vi "UHR-Fleezers Control (host) - 12.2.vi"() -> ()   [LabVIEW 2012] (continued)
      event "Green FB Setpoint (mV)", "Green FB Gains", "Green FB On/Off", "Current When FB OFF (%)", "Green int current ON count adj": Value Change {
        n2009 = event-data() -> ()  [unwired: 7 out]
        n2010 = local read "Green FB Setpoint (mV)"() -> (w3377:dbl)
        n2011 = Multiply(x=w3377, y=3.2767) -> (x*y=w3376:dbl)
        n2012 = local read "Current When FB OFF (%)"() -> (w3380:dbl)
        n2013 = Multiply(x=w3380, y=655.35) -> (x*y=w3381:dbl)
        n2014 = To Unsigned Word Integer(number=w3381) -> (unsigned 16bit integer=w3379:u16)
        n2015 = local read "Green int current ON count adj"() -> (w3383:u32)
        n2016 = local read "Green Laser ON/Interlacing"() -> (w3374:bool)
        n2017 = local read "Laser interlacing mode"() -> (w3373:enum32{"Laser ON", "Laser OFF", "Interlace"})
        n2018 = local read "Green FB Gains"() -> (w3370:T9)
        n2019 = local read "Green FB On/Off"() -> (w3384:bool)
        n2020 = Equal?(x=w3373, y=enum32{"Laser ON", "Laser OFF", "Interlace"}."Interlace") -> (x = y?=w3371:bool)
        n2021 = Unbundle By Name(w3370) -> ("proportional gain (Kc)"=w3369:i16, "integral gain (Kc*Ts/Ti)"=w3368:i16, "derivative gain (Kc*Td/Ts)"=w3367:i16)
        n2022 = Compound Arithmetic op=AND(w3371, w3384, w3374) -> (w3375:bool)
        n2023 = xnode "Read/Write Control"("FPGA VI Reference In"=w3387, "error in"=w3386, "Green FB Setpoint"=w3376, "Green FB On/Off"=w3375, "Current Out"=w3379, "Green int current ON count adj"=w3383, "P3"=w3369, "I3"=w3368, "D3"=w3367) -> ("error out"=w3385:errorcluster)  [unwired: 1 out]
      }
      event "Red FB Setpoint (mV)", "Red FB Gains", "Red FB On/Off", "Current When RI FB OFF (%)", "Red int current ON count adj": Value Change {
        n2024 = event-data() -> ()  [unwired: 7 out]
        n2025 = local read "Red FB Setpoint (mV)"() -> (w3399:dbl)
        n2026 = Multiply(x=w3399, y=3.2767) -> (x*y=w3398:dbl)
        n2027 = local read "Current When RI FB OFF (%)"() -> (w3388:dbl)
        n2028 = Multiply(x=w3388, y=655.35) -> (x*y=w3402:dbl)
        n2029 = To Unsigned Word Integer(number=w3402) -> (unsigned 16bit integer=w3401:u16)
        n2030 = local read "Red int current ON count adj"() -> (w3404:u32)
        n2031 = local read "Red Laser ON/Interlacing"() -> (w3396:bool)
        n2032 = local read "Laser interlacing mode"() -> (w3395:enum32{"Laser ON", "Laser OFF", "Interlace"})
        n2033 = local read "Red FB Gains"() -> (w3392:T9)
        n2034 = local read "Red FB On/Off"() -> (w3405:bool)
        n2035 = Equal?(x=w3395, y=enum32{"Laser ON", "Laser OFF", "Interlace"}."Interlace") -> (x = y?=w3393:bool)
        n2036 = Unbundle By Name(w3392) -> ("proportional gain (Kc)"=w3391:i16, "integral gain (Kc*Ts/Ti)"=w3390:i16, "derivative gain (Kc*Td/Ts)"=w3389:i16)
        n2037 = Compound Arithmetic op=AND(w3393, w3405, w3396) -> (w3397:bool)
        n2038 = xnode "Read/Write Control"("FPGA VI Reference In"=w3408, "error in"=w3407, "Red FB Setpoint"=w3398, "Red FB On/Off"=w3397, "RI Current Out"=w3401, "Red int current ON count adj"=w3404, "P4"=w3391, "I4"=w3390, "D4"=w3389) -> ("error out"=w3406:errorcluster)  [unwired: 1 out]
      }
      event "Laser interlacing mode", "Green Laser ON/Interlacing", "Red Laser ON/Interlacing": Value Change {
        n2039 = event-data() -> ()  [unwired: 7 out]
        n2040 = local write "Green Laser ON/OFF"("Green Laser ON/Interlacing") -> ()
        n2041 = local write "Red Laser ON/OFF"("Red Laser ON/Interlacing") -> ()
        n2042 = case shown="True" "Green Laser ON/Interlacing" {
          tunnel: "Laser interlacing mode" -> [_ w3432]
          tunnel: [enum32{"Laser ON", "Laser OFF", "Interlace"}."Laser OFF" ("Green laser mode") w3432] -> w3415
          tunnel: [FALSE w3428] -> w3414
          frame False {
          }
          frame True {
            n2043 = local read "Green FB On/Off"() -> (w3429:bool)
            n2044 = Equal?(x=w3432, y=enum32{"Laser ON", "Laser OFF", "Interlace"}."Interlace") -> (x = y?=w3430:bool)
            n2045 = And(x=w3430, y=w3429) -> (x .and. y?=w3428:bool)
          }
        }
        n2046 = case shown="True" "Red Laser ON/Interlacing" {
          tunnel: "Laser interlacing mode" -> [_ w3425]
          tunnel: [enum32{"Laser ON", "Laser OFF", "Interlace"}."Laser OFF" ("Green laser mode") w3425] -> w3410
          tunnel: [FALSE w3421] -> w3409
          frame False {
          }
          frame True {
            n2047 = local read "Red FB On/Off"() -> (w3422:bool)
            n2048 = Equal?(x=w3425, y=enum32{"Laser ON", "Laser OFF", "Interlace"}."Interlace") -> (x = y?=w3423:bool)
            n2049 = And(x=w3423, y=w3422) -> (x .and. y?=w3421:bool)
          }
        }
        n2050 = xnode "Read/Write Control"("FPGA VI Reference In"=w3418, "error in"=w3416, "Operating Mode"=w3415, "Operating Mode 2"=w3415, "Green FB On/Off"=w3414, "Red Laser Operating Mode"=w3410, "RI Operating Mode 2"=w3410, "Red FB On/Off"=w3409) -> ("error out"=w3417:errorcluster)  [unwired: 1 out]
      }
      event "Green Laser ON/OFF": Value Change {
        n2051 = event-data() -> ()  [unwired: 7 out]
        n2052 = property on="Green Laser ON/Interlacing" class="Bool (strict)"("Val(Sgnl)"="Green Laser ON/OFF") -> ()  [unwired: 2 in, 2 out]
      }
      event "Red Laser ON/OFF": Value Change {
        n2053 = event-data() -> ()  [unwired: 7 out]
        n2054 = property on="Red Laser ON/Interlacing" class="Bool (strict)"("Val(Sgnl)"="Red Laser ON/OFF") -> ()  [unwired: 2 in, 2 out]
      }
      event "Test ttrig": Value Change {
        n2055 = event-data() -> ()  [unwired: 7 out]
        n2056 = xnode "Read/Write Control"("FPGA VI Reference In"=w3438, "error in"=w3437, "TTrig?"=TRUE) -> ("error out"=w3436:errorcluster)  [unwired: 1 out]
      }
      event "Neg. TTrig FPGA": Value Change {
        n2057 = event-data() -> ()  [unwired: 7 out]
        n2058 = xnode "Read/Write Control"("FPGA VI Reference In"=w3442, "error in"=w3441, "TTrig Negate Pos"="Neg. TTrig FPGA") -> ()  [unwired: 2 out]
      }
      event "- phase (APD 1 Gate)", "+ phase (APD 1 Gate)": Value Change {
        n2059 = event-data() -> ()  [unwired: 7 out]
        n2060 = local read "Phase Adj. (APD 1 Gate)"() -> (w3443:i16)
        n2061 = Negate(x=w3443) -> (-x=w3451:i16)
        n2062 = Select(t=w3451, s="- phase (APD 1 Gate)", f=w3443) -> (s? t:f=w3450:i16)
        n2063 = Or(x="- phase (APD 1 Gate)", y="+ phase (APD 1 Gate)") -> (x .or. y?=w3446:bool)
        n2064 = xnode "Read/Write Control"("FPGA VI Reference In"=w3453, "error in"=w3452, "Phase count adjustment (APD 1 Gate)"=w3450) -> ("FPGA VI Reference Out"=w3448:T19, "error out"=w3449:errorcluster)
        n2065 = xnode "Read/Write Control"("FPGA VI Reference In"=w3448, "error in"=w3449, "+ phase (APD 1 Gate)"=w3446) -> ("error out"=w3447:errorcluster)  [unwired: 1 out]
      }
      event "+ phase (APD 2 Gate)", "- phase (APD 2 Gate)": Value Change {
        n2066 = event-data() -> ()  [unwired: 7 out]
        n2067 = local read "Phase Adj. (APD 2 Gate)"() -> (w3454:i16)
        n2068 = Negate(x=w3454) -> (-x=w3462:i16)
        n2069 = Select(t=w3462, s="- phase (APD 2 Gate)", f=w3454) -> (s? t:f=w3461:i16)
        n2070 = Or(x="- phase (APD 2 Gate)", y="+ phase (APD 2 Gate)") -> (x .or. y?=w3457:bool)
        n2071 = xnode "Read/Write Control"("FPGA VI Reference In"=w3464, "error in"=w3463, "Phase count adjustment (APD 2 Gate)"=w3461) -> ("FPGA VI Reference Out"=w3459:T19, "error out"=w3460:errorcluster)
        n2072 = xnode "Read/Write Control"("FPGA VI Reference In"=w3459, "error in"=w3460, "+ phase (APD 2 Gate)"=w3457) -> ("error out"=w3458:errorcluster)  [unwired: 1 out]
      }
      event "Phase Adj. (APD Acq)", "+ phase (APD Acq)", "- phase (APD Acq)": Value Change {
        n2073 = event-data() -> ()  [unwired: 7 out]
        n2074 = local read "Phase Adj. (APD Acq)"() -> (w3467:i16)
        n2075 = Negate(x=w3467) -> (-x=w3473:i16)
        n2076 = Select(t=w3473, s="+ phase (APD Acq)", f=w3467) -> (s? t:f=w3472:i16)
        n2077 = Or(x="+ phase (APD Acq)", y="- phase (APD Acq)") -> (x .or. y?=w3468:bool)
        n2078 = xnode "Read/Write Control"("FPGA VI Reference In"=w3475, "error in"=w3474, "Phase Count Adjustment (APD Acq)"=w3472) -> ("FPGA VI Reference Out"=w3470:T19, "error out"=w3471:errorcluster)
        n2079 = xnode "Read/Write Control"("FPGA VI Reference In"=w3470, "error in"=w3471, "+ phase (APD Acq)"=w3468) -> ("error out"=w3469:errorcluster)  [unwired: 1 out]
      }
      event "Phase adj. (GI)", "+ phase (GI)", "- phase (GI)", "Phase adj. (GI) 2", "+ phase (GI) 2", "- phase (GI) 2", "Phase adj. (RI)", "+ phase (RI)", "- phase (RI)", "Phase adj. (RI) 2", "+ phase (RI) 2", "- phase (RI) 2", "Phase adj. (Green FB)", "+ phase (Green FB)", "- phase (Green FB)", "Phase adj. (RI FB)", "+ phase (RI FB)", "- phase (RI FB)": Value Change {
        n2080 = event-data() -> ()  [unwired: 7 out]
        n2081 = Or(x="+ phase (GI)", y="- phase (GI)") -> (x .or. y?=w3509:bool)
        n2082 = Negate(x="Phase adj. (GI)") -> (-x=w3514:i16)
        n2083 = Select(t=w3514, s="+ phase (GI)", f="Phase adj. (GI)") -> (s? t:f=w3513:i16)
        n2084 = Or(x="+ phase (GI) 2", y="- phase (GI) 2") -> (x .or. y?=w3500:bool)
        n2085 = Negate(x="Phase adj. (GI) 2") -> (-x=w3505:i16)
        n2086 = Select(t=w3505, s="+ phase (GI) 2", f="Phase adj. (GI) 2") -> (s? t:f=w3501:i16)
        n2087 = Negate(x="Phase adj. (RI)") -> (-x=w3499:i16)
        n2088 = Or(x="+ phase (RI)", y="- phase (RI)") -> (x .or. y?=w3495:bool)
        n2089 = Select(t=w3499, s="+ phase (RI)", f="Phase adj. (RI)") -> (s? t:f=w3494:i16)
        n2090 = Negate(x="Phase adj. (RI) 2") -> (-x=w3493:i16)
        n2091 = Or(x="+ phase (RI) 2", y="- phase (RI) 2") -> (x .or. y?=w3482:bool)
        n2092 = Select(t=w3493, s="+ phase (RI) 2", f="Phase adj. (RI) 2") -> (s? t:f=w3489:i16)
        n2093 = Or(x="+ phase (Green FB)", y="- phase (Green FB)") -> (x .or. y?=w3483:bool)
        n2094 = Negate(x="Phase adj. (Green FB)") -> (-x=w3488:i16)
        n2095 = Select(t=w3488, s="+ phase (Green FB)", f="Phase adj. (Green FB)") -> (s? t:f=w3484:i16)
        n2096 = Or(x="+ phase (RI FB)", y="- phase (RI FB)") -> (x .or. y?=w3476:bool)
        n2097 = Negate(x="Phase adj. (RI FB)") -> (-x=w3481:i16)
        n2098 = Select(t=w3481, s="+ phase (RI FB)", f="Phase adj. (RI FB)") -> (s? t:f=w3477:i16)
        n2099 = xnode "Read/Write Control"("FPGA VI Reference In"=w3516, "error in"=w3515, "Phase count adjustment (GI)"=w3513, "Phase count adjustment (GI) 2"=w3501, "Phase count adjustment (RI)"=w3494, "Phase count adjustment (RI) 2"=w3489, "Phase count adjustment (Green FB)"=w3484, "Phase count adjustment (Red FB)"=w3477) -> ("FPGA VI Reference Out"=w3511:T19, "error out"=w3512:errorcluster)
        n2100 = xnode "Read/Write Control"("FPGA VI Reference In"=w3511, "error in"=w3512, "+ phase (GI)"=w3509, "+ phase (GI) 2"=w3500, "+ phase (RI)"=w3495, "+ phase (RI) 2"=w3482, "+ phase (Green FB)"=w3483, "+ phase (Red FB)"=w3476) -> ("error out"=w3510:errorcluster)  [unwired: 1 out]
      }
      event "Invert APD Gate", "APD Gate ON Count", "APD Gate OFF Count", "APD Gate", "APD Integration Time (s)", "APD 1 AO Mult.", "APD 2 AO Mult.", "Duty Cycles (ON one out of N cycles)": Value Change {
        n2101 = event-data() -> ()  [unwired: 7 out]
        n2102 = Add(x="Interlace Frequency, ON count", y="Interlace Frequency, OFF count") -> (x+y=w3521:u32)
        n2103 = Add(x="APD Gate ON Count", y="APD Gate OFF Count") -> (x+y=w3533:u32)
        n2104 = Multiply(x="Duty Cycles (ON one out of N cycles)", y=w3521) -> (x*y=w3517:u32)
        "Green FB Count" <- w3517
        "Red FB Count" <- w3517
        n2105 = Subtract(x=w3517, y="Interlace Frequency, ON count") -> (x-y=w3520:u32)
        n2106 = Multiply(x=w3533, y="Duty Cycles (ON one out of N cycles)") -> (x*y=w3532:u32)
        n2107 = Subtract(x=w3532, y="APD Gate ON Count") -> (x-y=w3531:u32)
        n2108 = local read "DMA Update Period (s)"() -> (w3534:dbl)
        n2109 = Multiply(x="APD Integration Time (s)", y=40000000.0) -> (x*y=w3539:dbl)
        n2110 = Reciprocal(x="APD Integration Time (s)") -> (1/x=→"APD Acq Rate (Hz)":dbl)
        n2111 = To Unsigned Long Integer(number=w3539) -> (unsigned 32bit integer=w3523:u32)
        "APD Int. Count" <- w3523
        n2112 = Divide(x=w3534, y="APD Integration Time (s)") -> (x/y=w3537:dbl)
        n2113 = Multiply(x=2.0, y=w3537) -> (x*y=w3536:dbl)
        n2114 = local write "APD Samples/FIFO Acq."(w3537) -> ()
        n2115 = xnode "Read/Write Control"("FPGA VI Reference In"=w3543, "error in"=w3542, "Invert APD Gate"="Invert APD Gate", "APD Gate ON Count"="APD Gate ON Count", "APD Gate OFF Count"=w3531, "APD Acq Rate Count"=w3523, "APD Gate Operating Mode"="APD Gate", "APD 1 AO scale factor"="APD 1 AO Mult.", "APD 2 AO scale factor"="APD 2 AO Mult.", "Green interlace ON count"="Interlace Frequency, ON count", "Green interlace OFF count"=w3520, "Green interlace ON count 2"="Interlace Frequency, ON count", "Green interlace OFF count 2"=w3520, "Green FB Count"=w3517, "Red interlace ON count"="Interlace Frequency, ON count", "Red interlace OFF count"="Interlace Frequency, OFF count", "Red FB Count"=w3517, "Red interlace ON count 2"="Interlace Frequency, ON count", "Red interlace OFF count 2"="Interlace Frequency, OFF count") -> ("error out"=w3541:errorcluster)  [unwired: 1 out]
        n2116 = local write "APD Elements/DMA read"(w3536) -> ()
      }
      event "Number of F/B Scans (AOD)", "Scan Speed (nm/s)", "Scan BD", "Initial delta (MHz)", "Step Size (nm)", "Scan Range (nm)": Value Change {
        w3605 = 123.0  # AOM cal (nm/MHz)
        n2117 = event-data() -> ()  [unwired: 7 out]
        n2118 = local read "BD 1 Frequency 1 (MHz)"() -> (w3588:dbl)
        n2119 = local read "AOM X Cal (nm/MHz)"() -> (w3580:dbl)
        n2120 = local read "X RF Frequency Limits (MHz)"() -> (w3592:T16)
        n2121 = local read "Y RF Frequency Limits (MHz)"() -> (w3589:T16)
        n2122 = local read "BD 2 Frequency 1 (MHz)"() -> (w3594:dbl)
        n2123 = Negate(x="Scan Range (nm)") -> (-x=w3558:dbl)
        n2124 = Divide(x=w3558, y=w3580) -> (x/y=w3562:dbl)
        n2125 = Select(t=w3592, s="Scan BD", f=w3589) -> (s? t:f=w3591:T16)
        n2126 = Select(t=w3588, s="Scan BD", f=w3594) -> (s? t:f=w3593:dbl)
        n2127 = Unbundle By Name(w3591) -> ("Maximum"=w3600:dbl, "Minimum"=w3599:dbl)
        n2128 = Add(x=w3562, y=w3593) -> (x+y=w3597:dbl)
        n2129 = Divide(x=w3558, y="Step Size (nm)") -> (x/y=w3577:dbl)
        n2130 = Divide(x="Step Size (nm)", y=w3580) -> (x/y=w3586:dbl)
        n2131 = Absolute Value(x=w3577) -> (abs(x)=w3561:dbl)
        n2132 = Sign(1:w3558) -> (0:w3559:dbl)
        n2133 = In Range and Coerce(upper limit=w3600, x=w3597, lower limit=w3599) -> (coerced(x)=w3596:dbl, In Range?=w3598:bool)
        n2134 = To Unsigned Quad Integer(1:w3561) -> (0:w3576:u64)
        "Scan steps (AOD)" <- w3576
        n2135 = call "IR AOM freq to word.vi"("Frequency In (MHz)"=w3586) -> ("Frequency Word Out (double)"=w3583:dbl)
        n2136 = Multiply(x=w3559, y=w3583) -> (x*y=w3560:dbl)
        n2137 = Subtract(x=w3597, y=w3596) -> (x-y=w3595:dbl)
        n2138 = To Quad Integer(1:w3560) -> (0:w3582:i64)
        "Incr. int (AOD)" <- w3582
        n2139 = Subtract(x=w3562, y=w3595) -> (x-y=w3581:dbl)
        "Scan Range (MHz)" <- w3581
        n2140 = Select(t=w3562, s=w3598, f=w3581) -> (s? t:f=w3601:dbl)
        n2141 = Multiply(x=w3581, y=w3580) -> (x*y=w3579:dbl)
        n2142 = Decrement(x=w3576) -> (x-1=w3629:u64)
        n2143 = Negate(x=w3579) -> (-x=w3575:dbl)
        n2144 = local write "Scan Range (nm)"(w3575) -> ()
        n2145 = Divide(x=w3601, y=w3629) -> (x/y=w3585:dbl)
        "Scan Increment (MHz)" <- w3585
        n2146 = call "IR AOM freq to word.vi"("Frequency In (MHz)"=w3585) -> ("Frequency Word Out (double)"=w3584:dbl)
        n2147 = Divide(x="Step Size (nm)", y="Scan Speed (nm/s)") -> (x/y=w3572:dbl)
        n2148 = To Quad Integer(1:w3584) -> ()  [unwired: 1 out]
        n2149 = local read "Number Interlace Sets"() -> (w3556:u8)
        n2150 = local read "AI Count (ticks)"() -> (w3557:u32)
        n2151 = local read "Total Counts (ticks)"() -> (w3555:u32)
        n2152 = local read "# Samples/trap"() -> (w3587:u32)
        n2153 = Multiply(x=w3557, y=w3556) -> (x*y=w3554:u32)
        n2154 = Divide(x=w3555, y=w3554) -> (x/y=w3553:dbl)
        n2155 = Select(t=w3588, s="Scan BD", f=w3594) -> (s? t:f=w3626:dbl)
        "Initial freq. (MHz)" <- w3626
        n2156 = Add(x=w3601, y=w3626) -> (x+y=→"Final freq. (MHz)":dbl)
        n2157 = Divide(x=w3555, y=40000000.0) -> (x/y=w3571:dbl)
        n2158 = Divide(x=w3572, y=w3571) -> (x/y=w3570:dbl)
        n2159 = To Unsigned Quad Integer(1:w3570) -> (0:w3545:u64)
        n2160 = Quotient & Remainder(x=w3545, y=u64 2) -> (x-y*floor(x/y)=w3549:u64)  [unwired: 1 out]
        n2161 = Equal?(x=w3549, y=u64 0) -> (x = y?=w3547:bool)
        n2162 = Decrement(x=w3545) -> (x-1=w3546:u64)
        n2163 = Select(t=w3545, s=w3547, f=w3546) -> (s? t:f=w3544:u64)
        "Cycles/step (AOD)" <- w3544
        n2164 = xnode "Read/Write Control"("FPGA VI Reference In"=w3637, "error in"=w3636, "Scan steps"=w3576, "Number of scans"="Number of F/B Scans (AOD)", "Cycles per step"=w3544, "Scan freq.  increment"=w3582, "Scan BD"="Scan BD") -> ("error out"=w3635:errorcluster)  [unwired: 1 out]
        n2165 = Multiply(x=w3576, y=w3544) -> (x*y=w3630:u64)
        n2166 = Multiply(x=w3630, y=u64 2) -> (x*y=w3552:u64)
        n2167 = Multiply(x=w3553, y=w3552) -> (x*y=w3551:dbl)
        "Data points/scan (f/b)" <- w3551
        n2168 = Multiply(x=w3551, y="Number of F/B Scans (AOD)") -> (x*y=w3633:dbl)
        "Data points/scans" <- w3633
        n2169 = Divide(x=w3633, y=w3587) -> (x/y=→"N sets should be saved":dbl)
        n2170 = Multiply(x=w3630, y=w3571) -> (x*y=w3569:dbl)
        "Time/Scan (s) (AOD)" <- w3569
        n2171 = Select(t=w3601, s="Scan BD", f=0.0) -> (s? t:f=w3627:dbl)
        n2172 = Select(t=0.0, s="Scan BD", f=w3601) -> (s? t:f=w3623:dbl)
        n2173 = local read "BD 2 Frequency 2 (MHz)"() -> (w3619:dbl)
        n2174 = local read "BD 1 Frequency 2 (MHz)"() -> (w3622:dbl)
        n2175 = Add(x=w3623, y=w3594) -> (x+y=w3620:dbl)
        n2176 = Add(x=w3588, y=w3627) -> (x+y=w3621:dbl)
        n2177 = Multiply(x=w3569, y=2.0) -> (x*y=w3568:dbl)
        n2178 = Multiply(x=w3568, y="Number of F/B Scans (AOD)") -> (x*y=w3565:dbl)
        n2179 = Divide(x=w3565, y=60.0) -> (x/y=→"Time to Finish All (min)":dbl)
        n2180 = Add(x="Trap 2 Bead Size (nm)", y="Trap 1 Bead Size (nm)") -> (x+y=w3609:dbl)
        n2181 = Divide(x=w3609, y=2.0) -> (x/y=w3603:dbl)
        n2182 = local read "Initial delta (MHz)"() -> (w3606:dbl)
        n2183 = Subtract(x=w3620, y=w3619) -> (x-y=w3617:dbl)
        n2184 = Subtract(x=w3621, y=w3622) -> (x-y=w3618:dbl)
        n2185 = Square(x=w3617) -> (x^2=w3616:dbl)
        n2186 = Square(x=w3618) -> (x^2=w3615:dbl)
        n2187 = Add(x=w3615, y=w3616) -> (x+y=w3614:dbl)
        n2188 = Square Root(x=w3614) -> (sqrt(x)=w3613:dbl)
        "Final delta (MHz)" <- w3613
        n2189 = Multiply(x=w3605, y=w3613) -> (x*y=w3612:dbl)
        n2190 = Multiply(x=w3606, y=w3605) -> (x*y=w3604:dbl)
        n2191 = Subtract(x=w3604, y=w3603) -> (x-y=→"Initial sep (nm)":dbl)
        n2192 = Subtract(x=w3612, y=w3603) -> (x-y=→"Final sep (nm)":dbl)
      }
      event "Freq or Amp switch first", "Swap F1 and F2", "Freq switch delay", "Amp switch delay": Value Change {
        n2193 = event-data() -> ()  [unwired: 7 out]
        n2194 = local read "Amp switch delay"() -> (w3638:u16)
        n2195 = local read "Swap F1 and F2"() -> (w3639:bool)
        n2196 = xnode "Read/Write Control"("FPGA VI Reference In"=w3642, "error in"=w3641, "Swap F1 and F2"=w3639, "Amp switch delay"=w3638) -> ("error out"=w3640:errorcluster)  [unwired: 1 out]
      }
      event "Scan steps (MCL)", "Number of scans (MCL)", "Scan Range (V)\n(of steps)", "2D or 1D Scan", "N APD Samp/step", "Fast Scan Dir", "Continuous MCL Scanning", "Scan lines (y)": Value Change {
        w3644 = 32767.0 ("y")
        n2197 = event-data() -> ()  [unwired: 7 out]
        n2198 = Select(t="Scan lines (y)", s="2D or 1D Scan", f="Number of scans (MCL)") -> (s? t:f=w3649:u64)
        n2199 = Decrement(x="Scan steps (MCL)") -> (x-1=w3665:u64)
        n2200 = Divide(x="Scan Range (V)\n(of steps)", y=w3665) -> (x/y=w3664:dbl)
        "Desired Scan Incr (V)" <- w3664
        n2201 = local read "APD Integration Time (s)"() -> (w3657:dbl)
        n2202 = Multiply(x=w3664, y=w3644) -> (x*y=w3673:dbl)
        n2203 = Divide(x=w3673, y=10.0) -> (x/y=w3663:dbl)
        "Desired incr (int)" <- w3663
        n2204 = local read "Update Count (MCL)"() -> (w3669:u32)
        n2205 = Round Toward -Infinity(1:w3663) -> (0:w3672:dbl)
        n2206 = To Word Integer(number=w3672) -> (16bit integer=w3647:i16)
        "Actual Incr. int (MCL)" <- w3647
        n2207 = Multiply(x=w3657, y=40000000.0) -> (x*y=w3670:dbl)
        n2208 = Divide(x=w3670, y=w3669) -> (x/y=w3668:dbl)
        n2209 = Multiply(x=i16 10, y=w3647) -> (x*y=w3645:i16)
        n2210 = Multiply(x="N APD Samp/step", y=w3668) -> (x*y=w3667:dbl)
        "Cycles/step (MCL)" <- w3667
        n2211 = Divide(x=w3645, y=w3644) -> (x/y=→"Actual MCL Inc (V)":dbl)
        n2212 = Multiply(x="N APD Samp/step", y="Scan steps (MCL)") -> (x*y=w3659:dbl)
        n2213 = local read "APD Samples/FIFO Acq."() -> (w3656:dbl)
        n2214 = Multiply(x=w3659, y=u64 2) -> (x*y=w3658:dbl)
        "Data points/scan (f+b)" <- w3658
        n2215 = Multiply(x=w3658, y=w3649) -> (x*y=w3676:dbl)
        "Data points/scans (MCL)" <- w3676
        n2216 = Multiply(x=w3657, y=w3658) -> (x*y=w3650:dbl)
        "Time/f+b scan (s) (MCL)" <- w3650
        n2217 = Divide(x=w3676, y=w3656) -> (x/y=→"N sets should be saved (MCL)":dbl)
        n2218 = Multiply(x=w3650, y=w3649) -> (x*y=→"Total Time (s)":dbl)
        n2219 = Not(x="Fast Scan Dir") -> (.not. x?=w3654:bool)
        n2220 = xnode "Read/Write Control"("FPGA VI Reference In"=w3680, "error in"=w3679, "Scan steps (MCL)"="Scan steps (MCL)", "Number of scans (MCL)"=w3649, "Cycles per step (MCL)"=w3667, "Scan freq.  increment (MCL)"=w3647, "1D or 2D Scan?"="2D or 1D Scan", "MCL Scan Axis"=w3654, "Cont. Scan (MCL)"="Continuous MCL Scanning") -> ("error out"=w3678:errorcluster)  [unwired: 1 out]
      }
      event "Read Cal": Value Change {
        w3682 = 1000.0 ("y")
        n2221 = event-data() -> ()  [unwired: 7 out]
        n2222 = local read "Save file name"() -> (w3707:path)
        n2223 = local write "Read Cal"(FALSE ("Read Cal")) -> ()
        n2224 = Strip Path(path=w3707) -> (stripped path=w3706:path)  [unwired: 1 out]
        n2225 = Path To String(path=w3706) -> (string=w3705:string)
        n2226 = Concatenate Strings(w3705, "\\current.cal" ("string")) -> (w3703:string)
        n2227 = String To Path(string=w3703) -> (path=w3702:path)
        n2228 = Open/Create/Replace File(file path (use dialog)=w3702, operation (0:open)=T35."open", access (0:read/write)=enum16{"read/write", "read-only", "write-only"}."read-only") -> (refnum out=w3710:refnum<file>, error out=w3696:errorcluster)  [unwired: 1 in, 3 out]
        n2229 = Deny Access(4:w3696, 7:w3710) -> (0:w3695:errorcluster, 3:w3701:refnum<file>)  [unwired: 1 out]
        n2230 = Read from Binary File(5:0.0, 8:w3695, 9:T36."big-endian, network order" ("byte order (0:big-endian, network order)"), 10:-1 ("count (1)"), 11:w3701) -> (0:w3694:errorcluster, 2:w3692:dbl[], 3:w3697:refnum<file>)  [unwired: 2 out]
        n2231 = Array To Cluster(array=w3692) -> (cluster=w3691:T44)
        n2232 = Unbundle(w3691) -> ("[0]"=w3690:dbl, "[1]"=w3689:dbl, "[2]"=w3688:dbl, "[3]"=w3687:dbl, "[4]"=w3686:dbl, "[5]"=w3685:dbl)
        n2233 = Close File(refnum=w3697, error in=w3694) -> (error out=→"Read cal error":errorcluster)  [unwired: 1 out]
        n2234 = Multiply(x=w3685, y=w3682) -> (x*y=w3683:dbl)
        n2235 = local write "T2 kappa_x (pN/nm)"(w3687) -> ()
        n2236 = local write "T1 kappa_x (pN/nm)"(w3688) -> ()
        n2237 = local write "T1 alpha_x (nm/V)"(w3690) -> ()
        n2238 = local write "T2 alpha_x (nm/V)"(w3689) -> ()
        n2239 = Multiply(x=w3686, y=w3682) -> (x*y=w3684:dbl)
        n2240 = local write "T1 offset_x (mV)"(w3684) -> ()
        n2241 = local write "T2 offset_x (mV)"(w3683) -> ()
      }
      event "Abort MCL Scan": Value Change {
        n2242 = event-data() -> ()  [unwired: 7 out]
        n2243 = local write "MCL Scanning"(FALSE ("MCL Scanning")) -> ()
        n2244 = xnode "Read/Write Control"("FPGA VI Reference In"=w3715, "error in"=w3714, "Abort scan (MCL)"="Abort MCL Scan") -> ("error out"=w3713:errorcluster)  [unwired: 1 out]
      }
      event "Update Count (MCL)": Value Change {
        n2245 = event-data() -> ()  [unwired: 7 out]
        n2246 = xnode "Read/Write Control"("FPGA VI Reference In"=w3719, "error in"=w3718, "MCL count"="Update Count (MCL)") -> ("error out"=w3717:errorcluster)  [unwired: 1 out]
      }
      event "Phase adjust (MCL)", "+ phase (MCL)", "- phase (MCL)": Value Change {
        n2247 = event-data() -> ()  [unwired: 7 out]
        n2248 = Negate(x="Phase adjust (MCL)") -> (-x=w3728:i16)
        n2249 = Select(t=w3728, s="- phase (MCL)", f="Phase adjust (MCL)") -> (s? t:f=w3726:i16)
        n2250 = Or(x="- phase (MCL)", y="+ phase (MCL)") -> (x .or. y?=w3721:bool)
        n2251 = xnode "Read/Write Control"("FPGA VI Reference In"=w3730, "error in"=w3729, "Phase count adjustment (MCL)"=w3726) -> ("FPGA VI Reference Out"=w3722:T19, "error out"=w3723:errorcluster)
        n2252 = xnode "Read/Write Control"("FPGA VI Reference In"=w3722, "error in"=w3723, "+ phase (MCL)"=w3721) -> ("error out"=w3720:errorcluster)  [unwired: 1 out]
      }
      event "Abort AOD Scan": Value Change {
        n2253 = event-data() -> ()  [unwired: 7 out]
        n2254 = xnode "Read/Write Control"("FPGA VI Reference In"=w3734, "error in"=w3733, "Abort scan"="Abort AOD Scan") -> ("error out"=w3732:errorcluster)  [unwired: 1 out]
      }
      event "Continuous AOD Scanning": Value Change {
        n2255 = event-data() -> ()  [unwired: 7 out]
        n2256 = xnode "Read/Write Control"("FPGA VI Reference In"=w3738, "error in"=w3737, "Cont. Scan"="Continuous AOD Scanning") -> ("error out"=w3736:errorcluster)  [unwired: 1 out]
      }
      event "Index": Value Change {
        n2257 = event-data() -> ()  [unwired: 7 out]
        n2258 = call "Create new save file.vi"("Insert"="", "Ext"=".dat" ("string"), "Index In"="Index") -> ("Path Out"=→"Save file name":path, "Index Out"=w3739:dbl)
        "Save index" <- w3739
        n2259 = local write "Index"(w3739) -> ()
      }
      event "AO1", "AO2": Value Change {
        w3754 = 10.0 ("y")
        w3753 = 32767.0 ("y")
        n2260 = event-data() -> ()  [unwired: 7 out]
        n2261 = local read "AO2"() -> (w3752:dbl)
        n2262 = local read "AO1"() -> (w3749:dbl)
        n2263 = Multiply(x=w3749, y=w3753) -> (x*y=w3748:dbl)
        n2264 = Multiply(x=w3752, y=w3753) -> (x*y=w3751:dbl)
        n2265 = Divide(x=w3748, y=w3754) -> (x/y=w3747:dbl)
        n2266 = Divide(x=w3751, y=w3754) -> (x/y=w3750:dbl)
        n2267 = To Word Integer(number=w3747) -> (16bit integer=w3755:i16)
        n2268 = To Word Integer(number=w3750) -> (16bit integer=w3756:i16)
        n2269 = xnode "Read/Write Control"("FPGA VI Reference In"=w3746, "error in"=w3745, "AO1"=w3755, "AO2"=w3756) -> ("error out"=w3744:errorcluster)  [unwired: 1 out]
      }
      event "Inject Pump 1": Value Change {
        n2270 = event-data() -> ()  [unwired: 7 out]
        n2271 = local read "Use Harvard pumps\nfor beads (else Chemyx)"() -> (w3758:bool)
        n2272 = case shown="True" w3758 {
          tunnel: "Inject Pump 1" -> [w3762 w3800]
          tunnel: w3757 -> [_ w3801]
          frame False {
            n2273 = local read "Pump write delay (ms)"() -> (w3761:dbl)
            n2274 = local read "Chemyx Syringe Pump Serial Port"() -> (w3760:refnum<visa-resource-name>)
            n2275 = case shown="True" w3762 {
              tunnel: w3761 -> [w3768 w3782]
              tunnel: w3760 -> [w3765 w3781]
              frame False {
                n2276 = flat-sequence {
                  tunnel: w3765 -> [w3769]
                  tunnel: [w3769] -> w3766
                  tunnel: w3768 -> [_]
                  tunnel: [w3772] -> w3767
                  tunnel: w3766 -> [w3772]
                  tunnel: w3767 -> [w3773]
                  tunnel: [w3773] -> w3763
                  tunnel: [w3775] -> w3764
                  tunnel: w3763 -> [w3775]
                  tunnel: w3764 -> [w3777]
                  frame #0 {
                    n2277 = call "Write to pump.vi"("string"="enter pump1", "VISA resource name"=w3769) -> ()  [unwired: 1 out]
                  }
                  frame #1 {
                    n2278 = Wait (ms)(milliseconds to wait="Pump pause delay (ms)") -> ()  [unwired: 1 out]
                  }
                  frame #2 {
                    n2279 = call "Write to pump.vi"("string"="stop", "VISA resource name"=w3773) -> ()  [unwired: 1 out]
                  }
                  frame #3 {
                    n2280 = Wait (ms)(milliseconds to wait=u32 500) -> ()  [unwired: 1 out]
                  }
                  frame #4 {
                    n2281 = call "Write to pump.vi"("string"="stop", "VISA resource name"=w3777) -> ()  [unwired: 1 out]
                  }
                }
              }
              frame True {
                n2282 = flat-sequence {
                  tunnel: w3781 -> [w3791]
                  tunnel: w3782 -> [w3786]
                  tunnel: w3782 -> [w3793]
                  tunnel: w3781 -> [w3794]
                  tunnel: [w3794] -> w3779
                  tunnel: [w3796] -> w3780
                  tunnel: w3779 -> [w3796]
                  tunnel: w3780 -> [w3798]
                  frame #0 {
                    n2283 = local read "All Pump Parameters"() -> (w3785:T5)
                    n2284 = Unbundle By Name(w3785) -> ("Pump 1"=w3792:T45)
                    n2285 = call "Set pump parameters.vi"("Pump write delay (ms)"=w3786, "Volume (uL)"="Ch 1 Inject Volume (uL)", "Rate (uL/h)"="Ch 1 Inject Rate (ul/h)", "Units"=4.0, "Pump #"=1.0, "Pump Parameters In"=w3792, "VISA resource name"=w3791) -> ("Pump Parameters Out"=w3784:T45)  [unwired: 3 in]
                    n2286 = Bundle By Name(cluster=w3785, "Pump 1"=w3784) -> (w3783:T5)
                    n2287 = local write "All Pump Parameters"(w3783) -> ()
                  }
                  frame #1 {
                    n2288 = Wait (ms)(milliseconds to wait=w3793) -> ()  [unwired: 1 out]
                  }
                  frame #2 {
                    n2289 = call "Write to pump.vi"("string"="start", "VISA resource name"=w3794) -> ()  [unwired: 1 out]
                  }
                  frame #3 {
                    n2290 = Wait (ms)(milliseconds to wait=u32 500) -> ()  [unwired: 1 out]
                  }
                  frame #4 {
                    n2291 = call "Write to pump.vi"("string"="start", "VISA resource name"=w3798) -> ()  [unwired: 1 out]
                  }
                }
              }
            }
          }
          frame True {
            n2292 = case shown="False" w3800 {
              tunnel: w3801 -> [w3802 w3812]
              frame False {
                n2293 = flat-sequence {
                  tunnel: w3802 -> [w3804]
                  frame #0 {
                    n2294 = local write "Flushing P1"(FALSE ("Flushing P1")) -> ()
                    n2295 = Concatenate Strings("stop" ("string"), "\r") -> (w3806:string)
                    n2296 = VISA Write(VISA resource name=w3804, write buffer=w3806) -> ()  [unwired: 1 in, 3 out]
                  }
                  frame #1 {
                    n2297 = property on="Clear Volume P1" class="Bool (strict)"("Val(Sgnl)"=TRUE ("Value (Signaling)")) -> ()  [unwired: 2 in, 2 out]
                  }
                }
              }
              frame True {
                n2298 = local read "Normal Flow Rate (ul/h) P1"() -> (w3810:dbl)
                n2299 = Number To Decimal String(number=w3810) -> (decimal integer string=w3816:string)  [unwired: 1 in]
                n2300 = Concatenate Strings("irate  " ("string"), w3816, " u/h" ("string"), "\r") -> (w3814:string)
                n2301 = VISA Write(VISA resource name=w3812, write buffer=w3814) -> (VISA resource name out=w3811:refnum<visa-resource-name>)  [unwired: 1 in, 2 out]
                n2302 = Concatenate Strings("irun" ("string"), "\r") -> (w3818:string)
                n2303 = VISA Write(VISA resource name=w3811, write buffer=w3818) -> ()  [unwired: 1 in, 3 out]
              }
            }
          }
        }
      }
      event "Inject Pump 3": Value Change {
        n2304 = event-data() -> ()  [unwired: 7 out]
        n2305 = local read "Use Harvard pumps\nfor beads (else Chemyx)"() -> (w3821:bool)
        n2306 = case shown="True" w3821 {
          tunnel: "Inject Pump 3" -> [w3825 w3864]
          tunnel: w3820 -> [_ w3863]
          frame False {
            n2307 = local read "Pump write delay (ms)"() -> (w3824:dbl)
            n2308 = case shown="True" w3825 {
              tunnel: w3824 -> [w3831 w3845]
              tunnel: "Chemyx Syringe Pump Serial Port" -> [w3828 w3844]
              frame False {
                n2309 = flat-sequence {
                  tunnel: w3828 -> [w3832]
                  tunnel: [w3832] -> w3829
                  tunnel: w3831 -> [_]
                  tunnel: [w3835] -> w3830
                  tunnel: w3829 -> [w3835]
                  tunnel: w3830 -> [w3836]
                  tunnel: [w3836] -> w3826
                  tunnel: [w3838] -> w3827
                  tunnel: w3826 -> [w3838]
                  tunnel: w3827 -> [w3840]
                  frame #0 {
                    n2310 = call "Write to pump.vi"("string"="enter pump3", "VISA resource name"=w3832) -> ()  [unwired: 1 out]
                  }
                  frame #1 {
                    n2311 = local read "Pump pause delay (ms)"() -> (w3834:u32)
                    n2312 = Wait (ms)(milliseconds to wait=w3834) -> ()  [unwired: 1 out]
                  }
                  frame #2 {
                    n2313 = call "Write to pump.vi"("string"="stop", "VISA resource name"=w3836) -> ()  [unwired: 1 out]
                  }
                  frame #3 {
                    n2314 = Wait (ms)(milliseconds to wait=u32 0) -> ()  [unwired: 1 out]
                  }
                  frame #4 {
                    n2315 = call "Write to pump.vi"("string"="stop", "VISA resource name"=w3840) -> ()  [unwired: 1 out]
                  }
                }
              }
              frame True {
                n2316 = flat-sequence {
                  tunnel: w3844 -> [w3854]
                  tunnel: w3845 -> [w3849]
                  tunnel: w3845 -> [w3856]
                  tunnel: w3844 -> [w3857]
                  tunnel: [w3857] -> w3843
                  tunnel: [w3860] -> w3842
                  tunnel: w3843 -> [w3860]
                  tunnel: w3842 -> [w3861]
                  frame #0 {
                    n2317 = local read "All Pump Parameters"() -> (w3848:T5)
                    n2318 = Unbundle By Name(w3848) -> ("Pump 3"=w3855:T45)
                    n2319 = call "Set pump parameters.vi"("Pump write delay (ms)"=w3849, "Volume (uL)"="Ch 3 Inject Volume (uL)", "Rate (uL/h)"="Ch 3 Inject Rate (ul/h)", "Units"=4.0, "Pump #"=3.0, "Pump Parameters In"=w3855, "VISA resource name"=w3854) -> ("Pump Parameters Out"=w3847:T45)  [unwired: 3 in]
                    n2320 = Bundle By Name(cluster=w3848, "Pump 3"=w3847) -> (w3846:T5)
                    n2321 = local write "All Pump Parameters"(w3846) -> ()
                  }
                  frame #1 {
                    n2322 = Wait (ms)(milliseconds to wait=w3856) -> ()  [unwired: 1 out]
                  }
                  frame #2 {
                    n2323 = call "Write to pump.vi"("string"="start", "VISA resource name"=w3857) -> ()  [unwired: 1 out]
                  }
                  frame #3 {
                    n2324 = Wait (ms)(milliseconds to wait=u32 500) -> ()  [unwired: 1 out]
                  }
                  frame #4 {
                    n2325 = call "Write to pump.vi"("string"="start", "VISA resource name"=w3861) -> ()  [unwired: 1 out]
                  }
                }
              }
            }
          }
          frame True {
            n2326 = case shown="False" w3864 {
              tunnel: w3863 -> [w3865 w3872]
              frame False {
                n2327 = flat-sequence {
                  tunnel: w3865 -> [w3867]
                  frame #0 {
                    n2328 = local write "Flushing P3"(FALSE ("Flushing P3")) -> ()
                    n2329 = Concatenate Strings("stop" ("string"), "\r") -> (w3869:string)
                    n2330 = VISA Write(VISA resource name=w3867, write buffer=w3869) -> ()  [unwired: 1 in, 3 out]
                  }
                  frame #1 {
                    n2331 = property on="Clear Volume P3" class="Bool (strict)"("Val(Sgnl)"=TRUE ("Value (Signaling)")) -> ()  [unwired: 2 in, 2 out]
                  }
                }
              }
              frame True {
                n2332 = local read "Normal Flow Rate (ul/h) P3"() -> (w3873:dbl)
                n2333 = Number To Decimal String(number=w3873) -> (decimal integer string=w3879:string)  [unwired: 1 in]
                n2334 = Concatenate Strings("irate  " ("string"), w3879, " u/h" ("string"), "\r") -> (w3877:string)
                n2335 = VISA Write(VISA resource name=w3872, write buffer=w3877) -> (VISA resource name out=w3875:refnum<visa-resource-name>)  [unwired: 1 in, 2 out]
                n2336 = Concatenate Strings("irun" ("string"), "\r") -> (w3881:string)
                n2337 = VISA Write(VISA resource name=w3875, write buffer=w3881) -> ()  [unwired: 1 in, 3 out]
              }
            }
          }
        }
      }
      event "Inject Pump 2": Value Change {
        n2338 = event-data() -> ()  [unwired: 7 out]
        n2339 = local read "Pump write delay (ms)"() -> (w3885:dbl)
        n2340 = flat-sequence {
          tunnel: w3883 -> [w3898]
          tunnel: w3885 -> [w3894]
          tunnel: "Inject Pump 2" -> [_]
          tunnel: w3885 -> [w3900]
          tunnel: w3883 -> [w3901]
          frame #0 {
            n2341 = local read "All Pump Parameters"() -> (w3893:T5)
            n2342 = Multiply(x=60.0, y="Flush Center Ch Rate (ul/m)") -> (x*y=w3890:dbl)
            n2343 = Unbundle By Name(w3893) -> ("Pump 2"=w3899:T45)
            n2344 = call "Set pump parameters.vi"("Pump write delay (ms)"=w3894, "Volume (uL)"="Flush Center Ch Volume (uL)", "Rate (uL/h)"=w3890, "Units"=3.0, "Pump #"=2.0, "Pump Parameters In"=w3899, "VISA resource name"=w3898) -> ("Pump Parameters Out"=w3892:T45)  [unwired: 3 in]
            n2345 = Bundle By Name(cluster=w3893, "Pump 2"=w3892) -> (w3891:T5)
            n2346 = local write "All Pump Parameters"(w3891) -> ()
            n2347 = Add(x="Flush Center Ch Volume (uL)", y="Total Volume\nFlushed (uL)") -> (x+y=w3887:dbl)
            n2348 = local write "Total Volume\nFlushed (uL)"(w3887) -> ()
          }
          frame #1 {
            n2349 = Wait (ms)(milliseconds to wait=w3900) -> ()  [unwired: 1 out]
          }
          frame #2 {
            n2350 = call "Write to pump.vi"("string"="start", "VISA resource name"=w3901) -> ()  [unwired: 1 out]
          }
        }
        n2351 = local read "Chemyx Syringe Pump Serial Port"() -> (w3883:refnum<visa-resource-name>)
      }
      event "Sample Channel\nFlow": Value Change {
        n2352 = event-data() -> ()  [unwired: 7 out]
        n2353 = Select(t="irun" ("string"), s="Sample Channel\nFlow", f="stop" ("string")) -> (s? t:f=w3905:string)
        n2354 = Concatenate Strings(w3905, "\r") -> (w3908:string)
        n2355 = VISA Write(VISA resource name=w3903, write buffer=w3908) -> ()  [unwired: 1 in, 3 out]
      }
      event "Start Flow": Value Change {
        n2356 = event-data() -> ()  [unwired: 7 out]
        n2357 = local write "Sample Channel\nFlow"(TRUE ("Sample Channel\nFlow")) -> ()
        n2358 = local write "Start Flow"(FALSE ("Start Flow")) -> ()
        n2359 = Concatenate Strings("irun" ("string"), "\r") -> (w3914:string)
        n2360 = VISA Write(VISA resource name=w3910, write buffer=w3914) -> ()  [unwired: 1 in, 3 out]
      }
      event "Stop Flow": Value Change {
        w3916 = FALSE ("Stop Flow")
        n2361 = event-data() -> ()  [unwired: 7 out]
        n2362 = local write "Stop Flow"(w3916) -> ()
        n2363 = local write "Sample Channel\nFlow"(w3916) -> ()
        n2364 = Concatenate Strings("stop" ("string"), "\r") -> (w3919:string)
        n2365 = VISA Write(VISA resource name=w3917, write buffer=w3919) -> ()  [unwired: 1 in, 3 out]
      }
      event "Flow rate (uL/h)": Value Change {
        n2366 = event-data() -> ()  [unwired: 7 out]
        n2367 = Number To Decimal String(number="Flow rate (uL/h)") -> (decimal integer string=w3926:string)  [unwired: 1 in]
        n2368 = Concatenate Strings("irate  " ("string"), w3926, " u/h" ("string"), "\r") -> (w3925:string)
        n2369 = VISA Write(VISA resource name=w3922, write buffer=w3925) -> ()  [unwired: 1 in, 3 out]
      }
      event "Flush Sample": Value Change {
        n2370 = event-data() -> ()  [unwired: 7 out]
        n2371 = flat-sequence {
          tunnel: w3931 -> [w3959]
          tunnel: [w3939] -> w3930
          tunnel: [w3933] -> w3928
          tunnel: w3930 -> [w3963]
          tunnel: [w3963] -> w3929
          tunnel: w3928 -> [w3962]
          tunnel: w3929 -> [w3968]
          frame #0 {
            # "set paramaters (rate, volume) for flush, clear volume"
            n2372 = Number To Decimal String(number="Flush rate (uL/m)") -> (decimal integer string=w3955:string)  [unwired: 1 in]
            n2373 = Concatenate Strings("irate  " ("string"), w3955, " u/m" ("string"), "\r") -> (w3957:string)
            n2374 = VISA Write(VISA resource name=w3959, write buffer=w3957) -> (VISA resource name out=w3953:refnum<visa-resource-name>)  [unwired: 1 in, 2 out]
            n2375 = Reciprocal(x="Flush rate (uL/m)") -> (1/x=w3936:dbl)
            n2376 = Number To Decimal String(number="Volume (uL)") -> (decimal integer string=w3944:string)  [unwired: 1 in]
            n2377 = Multiply(x="Volume (uL)", y=w3936) -> (x*y=w3935:dbl)
            n2378 = Concatenate Strings("tvolume  " ("string"), w3944, " u" ("string"), "\r") -> (w3942:string)
            n2379 = Multiply(x=w3935, y=60000.0) -> (x*y=w3933:dbl)
            n2380 = VISA Write(VISA resource name=w3953, write buffer=w3942) -> (VISA resource name out=w3941:refnum<visa-resource-name>)  [unwired: 1 in, 2 out]
            n2381 = Concatenate Strings("cvolume" ("string"), "\r") -> (w3940:string)
            n2382 = VISA Write(VISA resource name=w3941, write buffer=w3940) -> (VISA resource name out=w3951:refnum<visa-resource-name>)  [unwired: 1 in, 2 out]
            n2383 = Concatenate Strings("irun" ("string"), "\r") -> (w3949:string)
            n2384 = VISA Write(VISA resource name=w3951, write buffer=w3949) -> (VISA resource name out=w3939:refnum<visa-resource-name>)  [unwired: 1 in, 2 out]
          }
          frame #1 {
            # "Have to wait until\nflow is done to reset\nrate"
            n2385 = Add(x=w3962, y=100.0) -> (x+y=w3961:dbl)
            n2386 = Wait (ms)(milliseconds to wait=w3961) -> ()  [unwired: 1 out]
          }
          frame #2 {
            # "reset flow rate to usual flow rate"
            n2387 = local read "Flow rate (uL/h)"() -> (w3974:dbl)
            n2388 = Number To Decimal String(number=w3974) -> (decimal integer string=w3972:string)  [unwired: 1 in]
            n2389 = Concatenate Strings("irate  " ("string"), w3972, " u/h" ("string"), "\r") -> (w3970:string)
            n2390 = VISA Write(VISA resource name=w3968, write buffer=w3970) -> (VISA resource name out=w3964:refnum<visa-resource-name>)  [unwired: 1 in, 2 out]
            n2391 = Concatenate Strings("cvolume" ("string"), "\r") -> (w3965:string)
            n2392 = VISA Write(VISA resource name=w3964, write buffer=w3965) -> ()  [unwired: 1 in, 3 out]
          }
        }
      }
      event "Flush Pump 3": Value Change {
        n2393 = event-data() -> ()  [unwired: 7 out]
        n2394 = flat-sequence {
          tunnel: w3975 -> [w3978]
          frame #0 {
            # "set paramaters (rate, volume) for flush, clear volume"
            n2395 = Number To Decimal String(number="Flush rate (uL/m) P3") -> (decimal integer string=w4000:string)  [unwired: 1 in]
            n2396 = local write "Inject Pump 3"(TRUE ("Inject Pump 3")) -> ()
            n2397 = Concatenate Strings("irate  " ("string"), w4000, " u/m" ("string"), "\r") -> (w4002:string)
            n2398 = VISA Write(VISA resource name=w3978, write buffer=w4002) -> (VISA resource name out=w3998:refnum<visa-resource-name>)  [unwired: 1 in, 2 out]
            n2399 = Reciprocal(x="Flush rate (uL/m) P3") -> (1/x=w3982:dbl)
            n2400 = Number To Decimal String(number="Volume (uL) P3") -> (decimal integer string=w3989:string)  [unwired: 1 in]
            n2401 = Multiply(x="Volume (uL) P3", y=w3982) -> (x*y=w3981:dbl)
            n2402 = Concatenate Strings("tvolume  " ("string"), w3989, " u" ("string"), "\r") -> (w3987:string)
            n2403 = Multiply(x=w3981, y=60.0) -> (x*y=→"HP3 Flush Time (s)":dbl)
            n2404 = VISA Write(VISA resource name=w3998, write buffer=w3987) -> (VISA resource name out=w3986:refnum<visa-resource-name>)  [unwired: 1 in, 2 out]
            n2405 = Concatenate Strings("cvolume" ("string"), "\r") -> (w3985:string)
            n2406 = VISA Write(VISA resource name=w3986, write buffer=w3985) -> (VISA resource name out=w3996:refnum<visa-resource-name>)  [unwired: 1 in, 2 out]
            n2407 = Concatenate Strings("irun" ("string"), "\r") -> (w3994:string)
            n2408 = VISA Write(VISA resource name=w3996, write buffer=w3994) -> ()  [unwired: 1 in, 3 out]
          }
          frame #1 {
            "Flushing P3" <- TRUE ("Flushing P3")
          }
        }
      }
      event "Flush Pump 1": Value Change {
        n2409 = event-data() -> ()  [unwired: 7 out]
        n2410 = flat-sequence {
          tunnel: [w4016] -> w4006
          tunnel: w4005 -> [w4009]
          tunnel: w4006 -> [_]
          frame #0 {
            # "set paramaters (rate, volume) for flush, clear volume"
            n2411 = local write "Inject Pump 1"(TRUE ("Inject Pump 1")) -> ()
            n2412 = Number To Decimal String(number="Flush rate (uL/m) P1") -> (decimal integer string=w4032:string)  [unwired: 1 in]
            n2413 = Concatenate Strings("irate  " ("string"), w4032, " u/m" ("string"), "\r") -> (w4034:string)
            n2414 = VISA Write(VISA resource name=w4009, write buffer=w4034) -> (VISA resource name out=w4030:refnum<visa-resource-name>)  [unwired: 1 in, 2 out]
            n2415 = Reciprocal(x="Flush rate (uL/m) P1") -> (1/x=w4013:dbl)
            n2416 = Number To Decimal String(number="Volume (uL) P1") -> (decimal integer string=w4021:string)  [unwired: 1 in]
            n2417 = Multiply(x="Volume (uL) P1", y=w4013) -> (x*y=w4012:dbl)
            n2418 = Concatenate Strings("tvolume  " ("string"), w4021, " u" ("string"), "\r") -> (w4019:string)
            n2419 = Multiply(x=w4012, y=60.0) -> (x*y=→"HP1 Flush Time (s)":dbl)
            n2420 = VISA Write(VISA resource name=w4030, write buffer=w4019) -> (VISA resource name out=w4018:refnum<visa-resource-name>)  [unwired: 1 in, 2 out]
            n2421 = Concatenate Strings("cvolume" ("string"), "\r") -> (w4017:string)
            n2422 = VISA Write(VISA resource name=w4018, write buffer=w4017) -> (VISA resource name out=w4028:refnum<visa-resource-name>)  [unwired: 1 in, 2 out]
            n2423 = Concatenate Strings("irun" ("string"), "\r") -> (w4026:string)
            n2424 = VISA Write(VISA resource name=w4028, write buffer=w4026) -> (VISA resource name out=w4016:refnum<visa-resource-name>)  [unwired: 1 in, 2 out]
          }
          frame #1 {
            "Flushing P1" <- TRUE ("Flushing P3")
          }
        }
      }
      event "Clear Volume": Value Change {
        n2425 = event-data() -> ()  [unwired: 7 out]
        n2426 = Concatenate Strings("cvolume" ("string"), "\r") -> (w4038:string)
        n2427 = VISA Write(VISA resource name=w4037, write buffer=w4038) -> ()  [unwired: 1 in, 3 out]
      }
      event "Clear Volume P3": Value Change {
        n2428 = event-data() -> ()  [unwired: 7 out]
        n2429 = Concatenate Strings("cvolume" ("string"), "\r") -> (w4044:string)
        n2430 = VISA Write(VISA resource name=w4043, write buffer=w4044) -> ()  [unwired: 1 in, 3 out]
        n2431 = local write "Clear Volume P3"(FALSE ("Clear Volume P3")) -> ()
      }
      event "Clear Volume P1": Value Change {
        n2432 = event-data() -> ()  [unwired: 7 out]
        n2433 = Concatenate Strings("cvolume" ("string"), "\r") -> (w4049:string)
        n2434 = local write "Clear Volume P1"(FALSE ("Clear Volume P1")) -> ()
        n2435 = VISA Write(VISA resource name=w4048, write buffer=w4049) -> ()  [unwired: 1 in, 3 out]
      }
      event "Display On P3": Value Change {
        n2436 = event-data() -> ()  [unwired: 7 out]
        n2437 = Select(t="dim 100", s="Display On P3", f="dim 0") -> (s? t:f=w4055:string)
        n2438 = Concatenate Strings(w4055, "\r") -> (w4057:string)
        n2439 = VISA Write(VISA resource name=w4052, write buffer=w4057) -> ()  [unwired: 1 in, 3 out]
      }
      event "Display On P1": Value Change {
        n2440 = event-data() -> ()  [unwired: 7 out]
        n2441 = Select(t="dim 100", s="Display On P1", f="dim 0") -> (s? t:f=w4062:string)
        n2442 = Concatenate Strings(w4062, "\r") -> (w4064:string)
        n2443 = VISA Write(VISA resource name=w4059, write buffer=w4064) -> ()  [unwired: 1 in, 3 out]
      }
      event "Retract Pump 3": Value Change {
        n2444 = event-data() -> ()  [unwired: 7 out]
        n2445 = local write "Retract Pump 3"(FALSE ("Retract Pump 3")) -> ()
        n2446 = case shown="True" "Retract Pump 3" {
          tunnel: w4066 -> [_ w4069]
          frame False {
          }
          frame True {
            n2447 = Number To Decimal String(number="Retract Rate (uL/m)") -> (decimal integer string=w4087:string)  [unwired: 1 in]
            n2448 = Concatenate Strings("wrate  " ("string"), w4087, " u/m" ("string"), "\r") -> (w4089:string)
            n2449 = VISA Write(VISA resource name=w4069, write buffer=w4089) -> (VISA resource name out=w4080:refnum<visa-resource-name>)  [unwired: 1 in, 2 out]
            n2450 = Number To Decimal String(number="Retract Vol 3 (uL)") -> (decimal integer string=w4082:string)  [unwired: 1 in]
            n2451 = Concatenate Strings("tvolume  " ("string"), w4082, " u" ("string"), "\r") -> (w4079:string)
            n2452 = VISA Write(VISA resource name=w4080, write buffer=w4079) -> (VISA resource name out=w4075:refnum<visa-resource-name>)  [unwired: 1 in, 2 out]
            n2453 = Concatenate Strings("cvolume" ("string"), "\r") -> (w4076:string)
            n2454 = VISA Write(VISA resource name=w4075, write buffer=w4076) -> (VISA resource name out=w4070:refnum<visa-resource-name>)  [unwired: 1 in, 2 out]
            n2455 = Concatenate Strings("wrun" ("string"), "\r") -> (w4071:string)
            n2456 = VISA Write(VISA resource name=w4070, write buffer=w4071) -> ()  [unwired: 1 in, 3 out]
          }
        }
      }
      event "Retract Pump 1": Value Change {
        n2457 = event-data() -> ()  [unwired: 7 out]
        n2458 = local write "Retract Pump 1"(FALSE ("Retract Pump 1")) -> ()
        n2459 = case shown="True" "Retract Pump 1" {
          tunnel: w4091 -> [_ w4096]
          frame False {
          }
          frame True {
            n2460 = local read "Retract Rate (uL/m)"() -> (w4094:dbl)
            n2461 = Number To Decimal String(number=w4094) -> (decimal integer string=w4112:string)  [unwired: 1 in]
            n2462 = Concatenate Strings("wrate  " ("string"), w4112, " u/m" ("string"), "\r") -> (w4114:string)
            n2463 = VISA Write(VISA resource name=w4096, write buffer=w4114) -> (VISA resource name out=w4106:refnum<visa-resource-name>)  [unwired: 1 in, 2 out]
            n2464 = Number To Decimal String(number="Retract Vol 1 (uL)") -> (decimal integer string=w4108:string)  [unwired: 1 in]
            n2465 = Concatenate Strings("tvolume  " ("string"), w4108, " u" ("string"), "\r") -> (w4105:string)
